vi "Write HW cycle times.vi"(5 "Function":enum16{"Open file", "Write data", "Close File"}(ring), 7 "file path (use dialog)":path, 8 "error in (no error)":errorcluster, 9 "Ref Time Stamps in":u64[](array[numeric]), 10 "Image Time in":u64[](array[numeric]), 11 "HW Timings File":refnum<file>) -> (0 "error out":errorcluster, 3 "refnum out":refnum<file>)   [LabVIEW 2020]
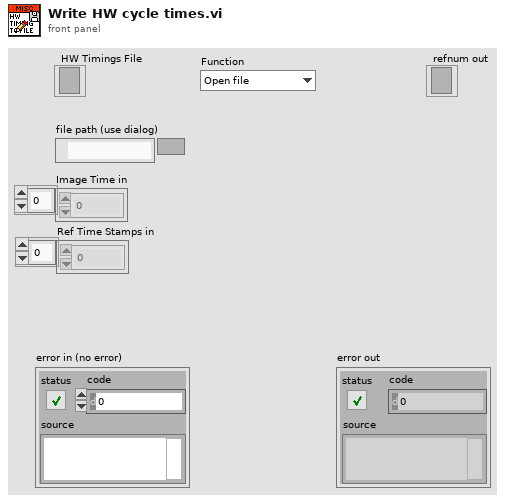
[diagram p1: front panel]
types:
  T1 = enum16{"open", "replace", "create", "open or create", "replace or create", "replace or create with confirmation"}
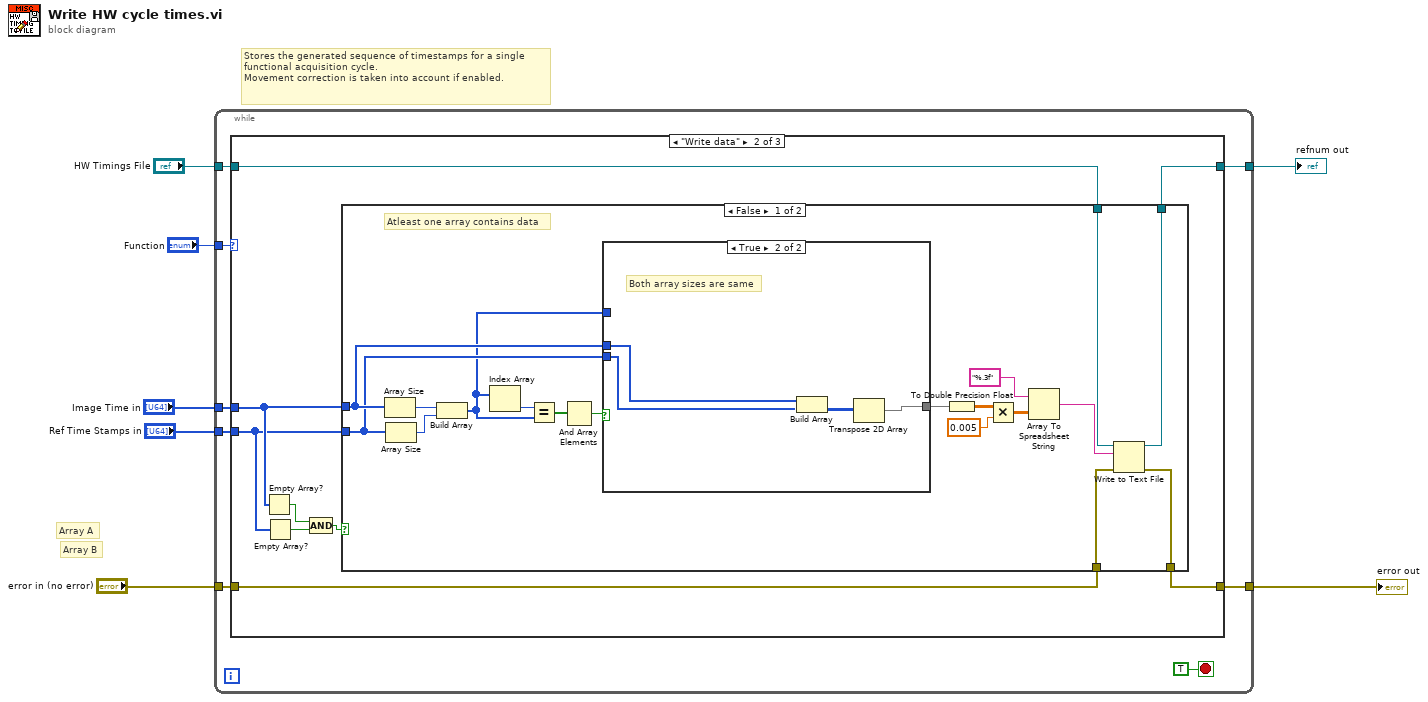
[diagram p0: block diagram]
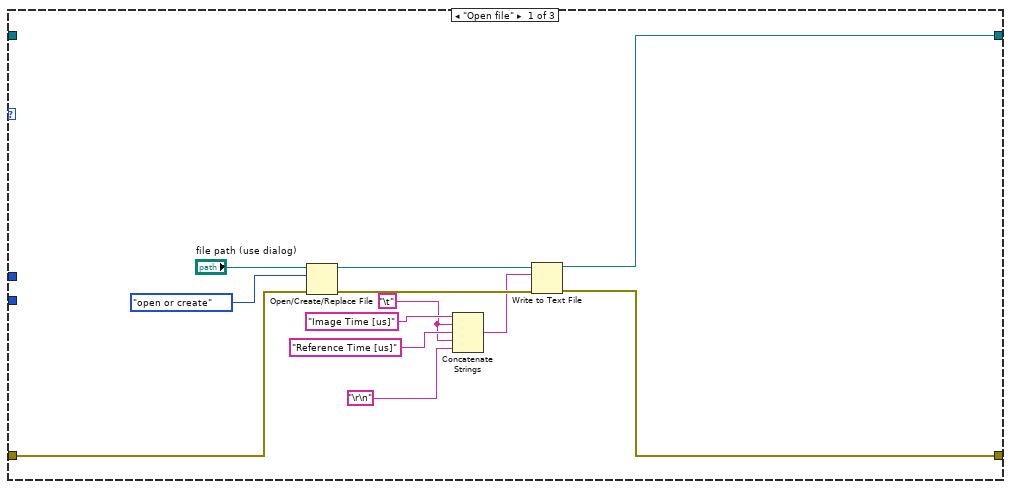
[diagram p2: hidden frame]
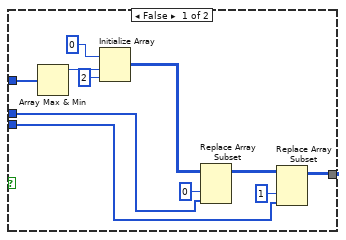
[diagram p3: hidden frame]
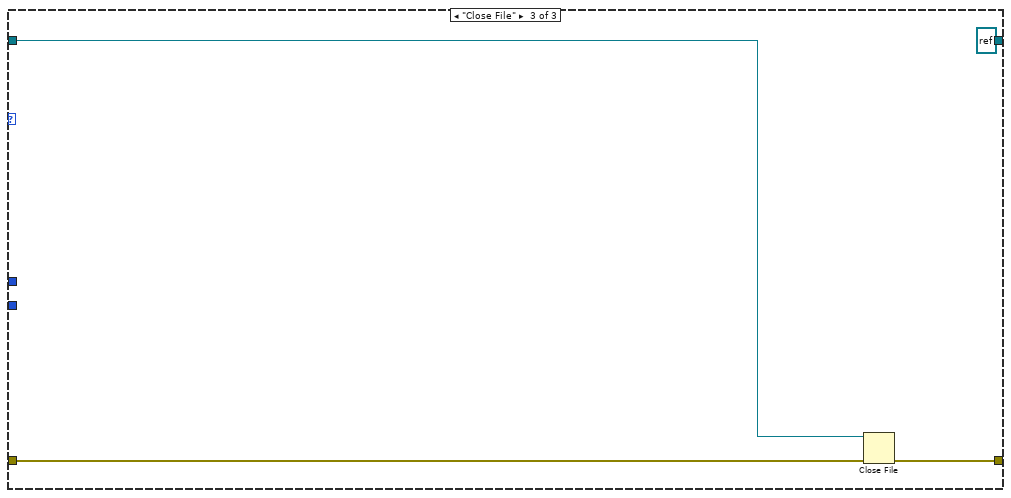
[diagram p5: hidden frame]
diagram:
  # "Array B"
  # "Array A"
  # "Stores the generated sequence of timestamps for a single functional acquisition cycle.\nMovement correction is taken into account if enabled."
  n1 = while {
    tunnel: "Image Time in" -> [w14]
    tunnel: "Function" -> [w13]
    tunnel: "error in (no error)" -> [w12]
    tunnel: [w11] -> w5
    tunnel: "Ref Time Stamps in" -> [w10]
    tunnel: "HW Timings File" -> [w9]
    tunnel: [w8] -> w3
    stop <- TRUE stop-if-true
    n2 = case shown="\"Write data\"" w13 {
      tunnel: w14 -> [_ w36 _]
      tunnel: w12 -> [w26 w34 w74]
      tunnel: [w18 w33 w75] -> w11
      tunnel: w10 -> [_ w35 _]
      tunnel: w9 -> [_ w32 w73]
      tunnel: [w19 w31 refnum<file> refnum ("HW Timings File")] -> w8
      frame "Open file" {
        w17 = "\t"
        n3 = Open/Create/Replace File(file path (use dialog)="file path (use dialog)", error in=w26, operation (0:open)=T1."open or create") -> (refnum out=w23:refnum<file>, error out=w24:errorcluster)  [unwired: 3 in, 1 out]
        n4 = Concatenate Strings("Image Time [us]", w17, "Reference Time [us]", w17, "\r\n") -> (w20:string)
        n5 = Write to Text File(file (use dialog)=w23, text=w20, error in=w24) -> (refnum out=w19:refnum<file>, error out=w18:errorcluster)  [unwired: 1 in, 1 out]
      }
      frame "Write data" {
        n6 = Empty Array?(array=w36) -> (empty?=w30:bool)
        n7 = Empty Array?(array=w35) -> (empty?=w29:bool)
        n8 = Compound Arithmetic op=AND(w30, w29) -> (w28:bool)
        n9 = case shown="False" w28 {
          tunnel: w36 -> [w54 _]
          tunnel: w35 -> [w40 _]
          tunnel: w34 -> [w49 w70]
          tunnel: [w48 w70] -> w33
          tunnel: w32 -> [w46 w71]
          tunnel: [w45 w71] -> w31
          frame False {
            # "Atleast one array contains data"
            n10 = Array Size(array=w54) -> (size(s)=w43:i32)
            n11 = Array Size(array=w40) -> (size(s)=w42:i32)
            n12 = Build Array(w43, w42) -> (w37:i32[])
            n13 = Index Array(array=w37) -> (element=w41:i32)  [unwired: 1 in]
            n14 = Equal?(x=w41, y=w37) -> (x = y?=w39:bool[])
            n15 = And Array Elements(Boolean array=w39) -> (logical AND=w38:bool)
            n16 = case shown="True" w38 {
              tunnel: w54 -> [w57 w69]
              tunnel: [w55 w67] -> w44
              tunnel: w40 -> [w56 w66]
              tunnel: w37 -> [w62 _]
              frame False {
                n17 = Array Max & Min(array=w62) -> (max value=w64:i32)  [unwired: 3 out]
                n18 = Initialize Array(u64 0 ("element"), w64, 2 ("dimension size")) -> (w58:u64[][])
                n19 = Replace Array Subset(array=w58, new element=w57, index (col)=0 ("disabled index (col)")) -> (w59:u64[][])  [unwired: 1 in]
                n20 = Replace Array Subset(array=w59, new element=w56, index (col)=1) -> (w55:u64[][])  [unwired: 1 in]
              }
              frame True {
                # "Both array sizes are same"
                n21 = Build Array(w69, w66) -> (w68:u64[][])
                n22 = Transpose 2D Array(2D array=w68) -> (transposed array=w67:u64[][])
              }
            }
            n23 = To Double Precision Float(number=w44) -> (double precision float=w53:dbl[][])
            n24 = Multiply(x=w53, y=0.005) -> (x*y=w51:dbl[][])
            n25 = Array To Spreadsheet String(array=w51, 3:"%.3f" ("format string")) -> (spreadsheet string=w47:string)  [unwired: 1 in]
            n26 = Write to Text File(file (use dialog)=w46, text=w47, error in=w49) -> (refnum out=w45:refnum<file>, error out=w48:errorcluster)  [unwired: 1 in, 1 out]
          }
          frame True {
            # "Arrays are empty"
          }
        }
      }
      frame "Close File" {
        n27 = Close File(refnum=w73, error in=w74) -> (error out=w75:errorcluster)  [unwired: 1 out]
      }
    }
  }
  "error out" <- w5
  "refnum out" <- w3
